vi "Assign Value.vi"(8 "error in (no error)":errorcluster, 10 "Assigned Value":refnum<class "Abs_Value.lvclass">, 11 "Abs_Variant in":refnum<class "Abs_Variant.lvclass">) -> (0 "error out":errorcluster, 3 "Abs_Variant out":refnum<class "Abs_Variant.lvclass">)   [LabVIEW 2021, in "Abs_Variant.lvclass"]
uses:
  Abs_Variant.lvclass
  Value/Abs_Value.lvclass
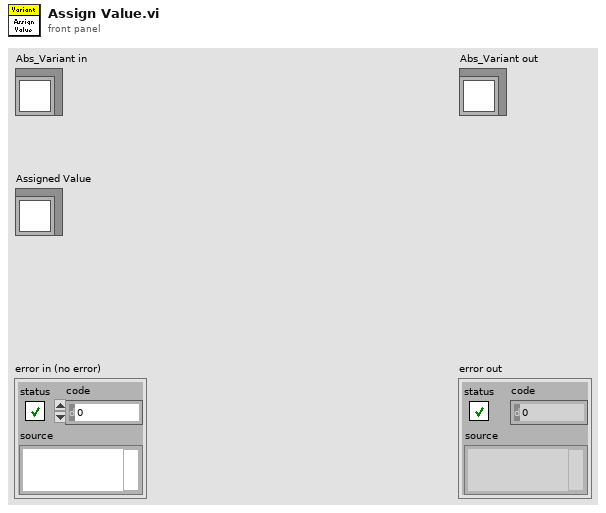
[diagram p1: front panel]
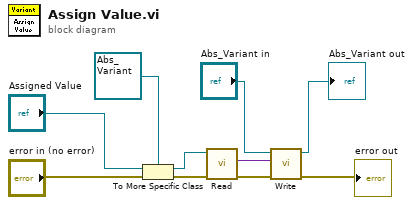
[diagram p0: block diagram]
diagram:
  n1 = To More Specific Class(target class=refnum<class "Abs_Variant.lvclass"> refnum ("Abs_Variant in"), reference="Assigned Value", error in="error in (no error)") -> (specific class reference=w6:refnum<class "Abs_Variant.lvclass">, error out=w7:errorcluster)
  n2 = call-dynamic "Read.vi"("error in (no error)"=w7, "Abs_Variant in"=w6) -> ("error out"=w5:errorcluster, "Variant"=w4:variant)  [unwired: 7 in, 1 out]
  n3 = call-dynamic "Write.vi"("error in (no error)"=w5, "Variant"=w4, "Abs_Variant in"="Abs_Variant in") -> ("error out"=→"error out":errorcluster, "Abs_Variant out"=→"Abs_Variant out":refnum<class "Abs_Variant.lvclass">)  [unwired: 7 in]
